vi "CRYCalc Arithmetic Unit&Ref.vi"(0 "A data for units":T1={"Name"="", "Curve"=[], "X data"=1, "Y data"=1, "Z data"=1, "X axis"=0, "Y axis"=1, "Z axis"=1, "X unit"="Hz", "Y unit"="", "Z unit"="deg.", "X dB ref"=1.0, "Y dB ref"=1.0, "Z dB ref"=1.0, "single val"=FALSE, "protected"=FALSE, "display X"=TRUE, "display Y"=TRUE, "display Z"=TRUE, "Test Info"="", "Step No."=0, "Plot Settings"={"Color"=0, "Interpolation"=0, "Point Style"=0, "Line Style"=0, "Point Color"=0, "Line Width"=0, "Bar Plot Style"=0, "Fill To"=0}, "AutoProtect"=FALSE} {"Z data" items=["dB", "Lin"]; "X data" items=["dB", "Lin"]; "Y data" items=["dB", "Lin"]; "Z dB ref" format="%.1f"; "Z axis" items=["Log", "Lin"]; "X dB ref" format="%.1f"; "X axis" items=["Log", "Lin"]; "Y axis" items=["Log", "Lin"]; "Y dB ref" format="%.1f"; "Curve"."z" format="%.2f"; "Curve"."y" format="%.2f"; "Curve"."x" format="%.2f"}, 5 "B data for units":T1={"Name"="", "Curve"=[], "X data"=1, "Y data"=1, "Z data"=1, "X axis"=0, "Y axis"=1, "Z axis"=1, "X unit"="Hz", "Y unit"="", "Z unit"="deg.", "X dB ref"=1.0, "Y dB ref"=1.0, "Z dB ref"=1.0, "single val"=FALSE, "protected"=FALSE, "display X"=TRUE, "display Y"=TRUE, "display Z"=TRUE, "Test Info"="", "Step No."=0, "Plot Settings"={"Color"=0, "Interpolation"=0, "Point Style"=0, "Line Style"=0, "Point Color"=0, "Line Width"=0, "Bar Plot Style"=0, "Fill To"=0}, "AutoProtect"=FALSE} {"Z data" items=["dB", "Lin"]; "X data" items=["dB", "Lin"]; "Y data" items=["dB", "Lin"]; "Z dB ref" format="%.1f"; "Z axis" items=["Log", "Lin"]; "X dB ref" format="%.1f"; "X axis" items=["Log", "Lin"]; "Y axis" items=["Log", "Lin"]; "Y dB ref" format="%.1f"; "Curve"."z" format="%.2f"; "Curve"."y" format="%.2f"; "Curve"."x" format="%.2f"}, 9 "operator":u16(ring) items=["+", "--", "x", "/"], 11 "Work in":u16(slide), 12 "Axis Mode":u16(slide)) -> (3 "Result X unit":string, 4 "Result Y unit":string, 6 "Result dB ref(A)":dbl=1.0 format="%.1f", 8 "Result Y data":u16, 10 "Single val out":bool, 14 "Result Z unit":string)   [LabVIEW 2013]
uses:
  Typedef Control/CRYData Cluster.ctl
  CRYPost Processing Global.vi
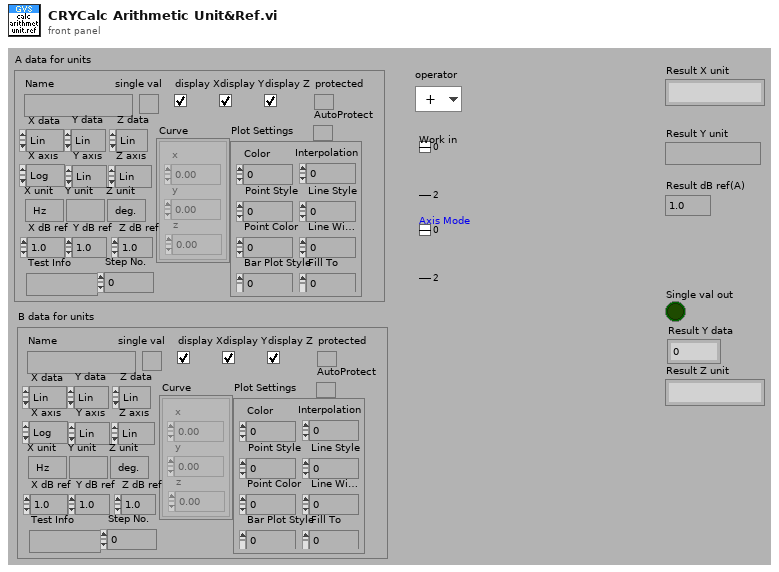
[diagram p1: front panel]
types:
  T1 = typedef "CRYData Cluster.ctl" = cluster{"Name":string, "Curve":cluster{"x":dbl, "y":dbl, "z":dbl}[], "X data":u16, "Y data":u16, "Z data":u16, "X axis":u16, "Y axis":u16, "Z axis":u16, "X unit":string, "Y unit":string, "Z unit":string, "X dB ref":dbl, "Y dB ref":dbl, "Z dB ref":dbl, "single val":bool, "protected":bool, "display X":bool, "display Y":bool, "display Z":bool, "Test Info":string, "Step No.":i32, "Plot Settings":cluster{"Color":u32, "Interpolation":u8, "Point Style":u8, "Line Style":u8, "Point Color":u32, "Line Width":u8, "Bar Plot Style":u8, "Fill To":i16}, "AutoProtect":bool}
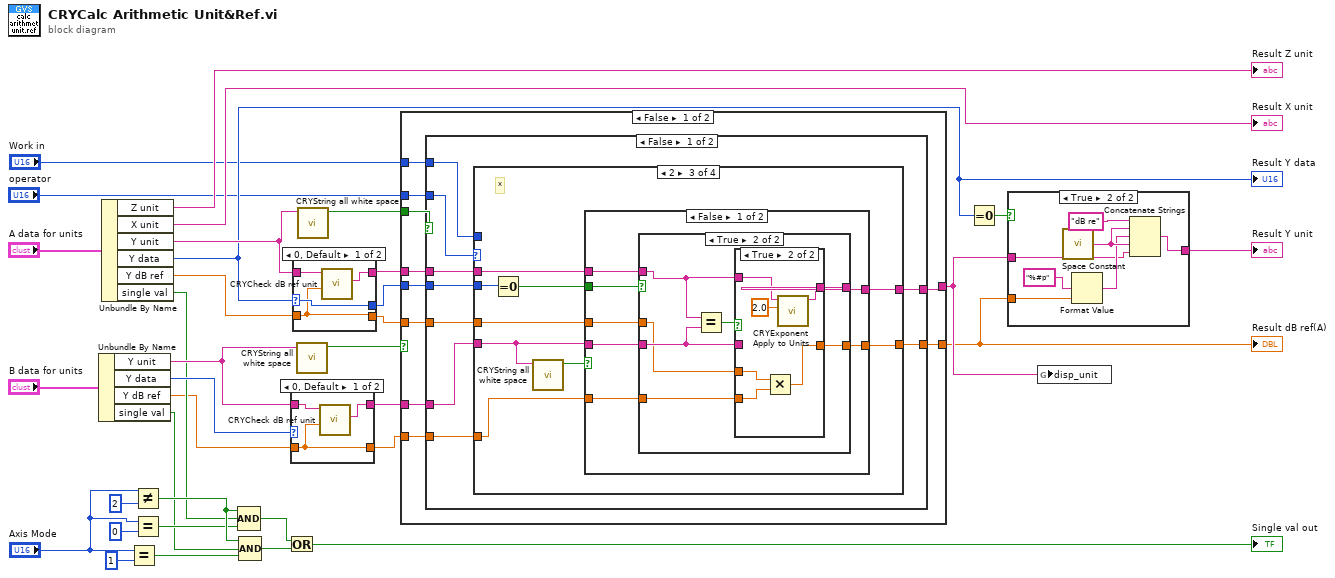
[diagram p0: block diagram]
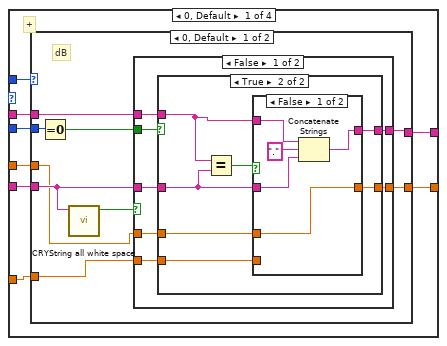
[diagram p2: hidden frame]
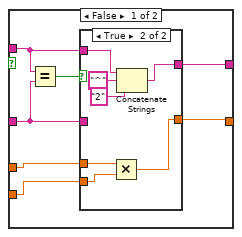
[diagram p3: hidden frame]
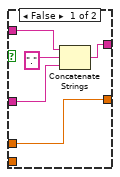
[diagram p4: hidden frame]
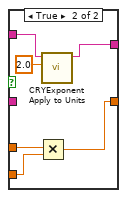
[diagram p5: hidden frame]
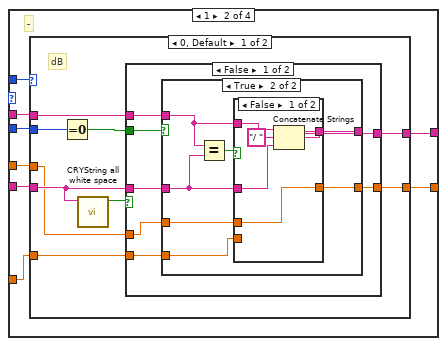
[diagram p8: hidden frame]
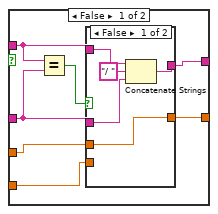
[diagram p9: hidden frame]
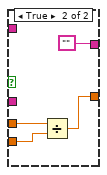
[diagram p10: hidden frame]
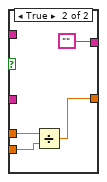
[diagram p11: hidden frame]
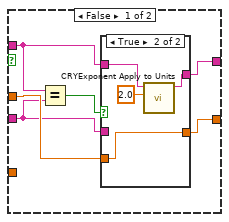
[diagram p14: hidden frame]
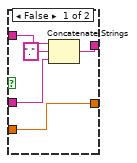
[diagram p15: hidden frame]
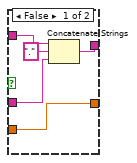
[diagram p16: hidden frame]
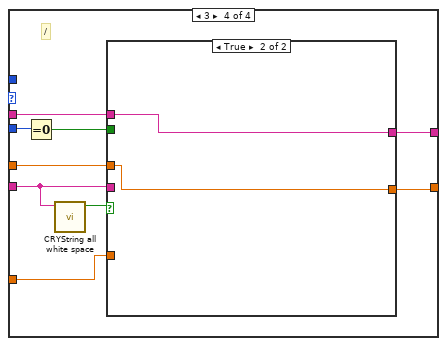
[diagram p18: hidden frame]
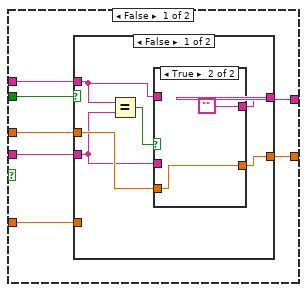
[diagram p19: hidden frame]
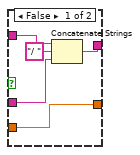
[diagram p20: hidden frame]
diagram:
  n1 = Unbundle By Name("B data for units") -> ("Y unit"=w35:string, "Y data"=w34:u16, "Y dB ref"=w17:dbl, "single val"=w21:bool)
  n2 = Unbundle By Name("A data for units") -> ("Z unit"=→"Result Z unit":string, "X unit"=→"Result X unit":string, "Y unit"=w14:string, "Y data"=w13:u16, "Y dB ref"=w12:dbl, "single val"=w22:bool)
  "Result Y data" <- w13
  n3 = Equal?(x="Axis Mode", y=u16 1) -> (x = y?=w28:bool)
  n4 = Not Equal?(x="Axis Mode", y=u16 2) -> (x != y?=w25:bool)
  n5 = Equal?(x="Axis Mode", y=u16 0) -> (x = y?=w23:bool)
  n6 = Compound Arithmetic op=AND(w25, w22, w23) -> (w26:bool)
  n7 = Compound Arithmetic op=AND(w25, w21, w28) -> (w27:bool)
  n8 = Or(x=w26, y=w27) -> (x .or. y?=→"Single val out":bool)
  n9 = case shown="0, Default" w34 {
    tunnel: w35 -> [w38 w40]
    tunnel: [w37 w40] -> w4
    tunnel: w17 -> [w36 w39]
    tunnel: [w36 w39] -> w1
    frame 0, Default {
      n10 = call "CRYCheck dB ref unit.vi"("dB ref in"=w36, "Unit in"=w38) -> ("Lin unit out"=w37:string)  [unwired: 9 out]
    }
    frame 1 {
    }
  }
  n11 = case shown="0, Default" w13 {
    selector: w13 -> [w42 w46]
    tunnel: w14 -> [w44 w47]
    tunnel: [w43 w47] -> w8
    tunnel: w12 -> [w41 w45]
    tunnel: [w42 w46] -> w7
    tunnel: [w41 w45] -> w6
    frame 0, Default {
      n12 = call "CRYCheck dB ref unit.vi"("dB ref in"=w41, "Unit in"=w44) -> ("Lin unit out"=w43:string)  [unwired: 9 out]
    }
    frame 1 {
    }
  }
  n13 = call "CRYString all white space.vi"("String"=w35) -> ("Nothing but white space?"=w5:bool)  [unwired: 10 in]
  n14 = call "CRYString all white space.vi"("String"=w14) -> ("Nothing but white space?"=w9:bool)  [unwired: 10 in]
  n15 = case shown="False" w5 {
    tunnel: [w57 w293] -> w3
    tunnel: w4 -> [w56 _]
    tunnel: w9 -> [w55 _]
    tunnel: w8 -> [w54 w293]
    tunnel: "Work in" -> [w53 _]
    tunnel: "operator" -> [w52 _]
    tunnel: w7 -> [w51 _]
    tunnel: w6 -> [w50 w292]
    tunnel: [w49 w292] -> w2
    tunnel: w1 -> [w48 _]
    frame False {
      n16 = case shown="False" w55 {
        tunnel: [w60 w291] -> w57
        tunnel: w56 -> [w63 w291]
        tunnel: w54 -> [w64 _]
        tunnel: w53 -> [w65 _]
        tunnel: w52 -> [w66 _]
        tunnel: w51 -> [w62 _]
        tunnel: w50 -> [w61 w290]
        tunnel: [w59 w290] -> w49
        tunnel: w48 -> [w58 _]
        frame False {
          n17 = case shown="2" w66 {
            tunnel: w65 -> [w74 w139 _ _]
            tunnel: w64 -> [w73 w138 w200 w251]
            tunnel: w63 -> [w72 w135 w196 w247]
            tunnel: w62 -> [w71 w137 w199 w250]
            tunnel: [w70 w134 w198 w249] -> w60
            tunnel: w61 -> [w69 w136 w194 w245]
            tunnel: [w68 w133 w192 w243] -> w59
            tunnel: w58 -> [w67 w132 w193 w244]
            frame 0, Default {
              # "+"
              n18 = case shown="0, Default" w74 {
                tunnel: w73 -> [w82 w131]
                tunnel: w72 -> [w79 _]
                tunnel: w71 -> [w83 _]
                tunnel: [w81 w131] -> w70
                tunnel: w69 -> [w76 w130]
                tunnel: [w75 w130] -> w68
                tunnel: w67 -> [w77 _]
                frame 0, Default {
                  # "dB"
                  n19 = Equal To 0?(x=w83) -> (x = 0?=w80:bool)
                  n20 = call "CRYString all white space.vi"("String"=w79) -> ("Nothing but white space?"=w78:bool)  [unwired: 10 in]
                  n21 = case shown="False" w78 {
                    tunnel: w82 -> [w90 w129]
                    tunnel: [w89 w129] -> w81
                    tunnel: w80 -> [w88 _]
                    tunnel: w79 -> [w87 _]
                    tunnel: w77 -> [w86 _]
                    tunnel: w76 -> [w85 w128]
                    tunnel: [w84 w128] -> w75
                    frame False {
                      n22 = case shown="True" w88 {
                        tunnel: w90 -> [w96 w113]
                        tunnel: w87 -> [w94 w114]
                        tunnel: [w95 w115] -> w89
                        tunnel: w86 -> [w92 w111]
                        tunnel: w85 -> [w93 w112]
                        tunnel: [w91 w110] -> w84
                        frame False {
                          n23 = Equal?(x=w96, y=w94) -> (x = y?=w97:bool)
                          n24 = case shown="True" w97 {
                            tunnel: w96 -> [w102 w109]
                            tunnel: [w99 w106] -> w95
                            tunnel: w94 -> [w100 _]
                            tunnel: w93 -> [w98 w105]
                            tunnel: w92 -> [_ w104]
                            tunnel: [w98 w103] -> w91
                            frame False {
                              n25 = Concatenate Strings(w102, "." ("string"), w100) -> (w99:string)
                            }
                            frame True {
                              n26 = Multiply(x=w105, y=w104) -> (x*y=w103:dbl)
                              n27 = Concatenate Strings(w109, "^" ("string"), "2" ("string")) -> (w106:string)
                            }
                          }
                        }
                        frame True {
                          n28 = Equal?(x=w113, y=w114) -> (x = y?=w116:bool)
                          n29 = case shown="False" w116 {
                            tunnel: w113 -> [w119 w126]
                            tunnel: [w118 w125] -> w115
                            tunnel: w114 -> [w120 _]
                            tunnel: w112 -> [w117 w124]
                            tunnel: w111 -> [_ w123]
                            tunnel: [w117 w122] -> w110
                            frame False {
                              n30 = Concatenate Strings(w119, "." ("string"), w120) -> (w118:string)
                            }
                            frame True {
                              n31 = Multiply(x=w124, y=w123) -> (x*y=w122:dbl)
                              n32 = call "CRYExponent Apply to Units.vi"("Exponent to apply"=2.0, "Unit in"=w126) -> ("Unit out"=w125:string)  [unwired: 9 out]
                            }
                          }
                        }
                      }
                    }
                    frame True {
                    }
                  }
                }
                frame 1, 2 {
                }
              }
            }
            frame 1 {
              # "-"
              n33 = case shown="0, Default" w139 {
                tunnel: w138 -> [w147 w191]
                tunnel: w135 -> [w144 _]
                tunnel: w137 -> [w148 _]
                tunnel: [w146 w191] -> w134
                tunnel: w136 -> [w142 w190]
                tunnel: [w140 w190] -> w133
                tunnel: w132 -> [w141 _]
                frame 0, Default {
                  # "dB"
                  n34 = Equal To 0?(x=w148) -> (x = 0?=w145:bool)
                  n35 = call "CRYString all white space.vi"("String"=w144) -> ("Nothing but white space?"=w143:bool)  [unwired: 10 in]
                  n36 = case shown="False" w143 {
                    tunnel: w147 -> [w155 w189]
                    tunnel: [w154 w189] -> w146
                    tunnel: w145 -> [w153 _]
                    tunnel: w144 -> [w152 _]
                    tunnel: w142 -> [w151 w188]
                    tunnel: w141 -> [w150 _]
                    tunnel: [w149 w188] -> w140
                    frame False {
                      n37 = case shown="True" w153 {
                        tunnel: w155 -> [w161 w175]
                        tunnel: w152 -> [w160 w176]
                        tunnel: [w159 w177] -> w154
                        tunnel: w151 -> [w158 w174]
                        tunnel: w150 -> [w157 w173]
                        tunnel: [w156 w172] -> w149
                        frame False {
                          n38 = Equal?(x=w161, y=w160) -> (x = y?=w162:bool)
                          n39 = case shown="False" w162 {
                            tunnel: w161 -> [w166 _]
                            tunnel: [w167 ""] -> w159
                            tunnel: w160 -> [w164 _]
                            tunnel: w158 -> [w163 w170]
                            tunnel: w157 -> [_ w169]
                            tunnel: [w163 w168] -> w156
                            frame False {
                              n40 = Concatenate Strings(w166, "/ " ("string"), w164) -> (w167:string)
                            }
                            frame True {
                              n41 = Divide(x=w170, y=w169) -> (x/y=w168:dbl)
                            }
                          }
                        }
                        frame True {
                          n42 = Equal?(x=w175, y=w176) -> (x = y?=w178:bool)
                          n43 = case shown="False" w178 {
                            tunnel: w175 -> [w182 _]
                            tunnel: [w183 ""] -> w177
                            tunnel: w176 -> [w180 _]
                            tunnel: w174 -> [w179 w186]
                            tunnel: w173 -> [_ w185]
                            tunnel: [w179 w184] -> w172
                            frame False {
                              n44 = Concatenate Strings(w182, "/ " ("string"), w180) -> (w183:string)
                            }
                            frame True {
                              n45 = Divide(x=w186, y=w185) -> (x/y=w184:dbl)
                            }
                          }
                        }
                      }
                    }
                    frame True {
                    }
                  }
                }
                frame 1, 2 {
                }
              }
            }
            frame 2 {
              # "*"
              n46 = Equal To 0?(x=w199) -> (x = 0?=w197:bool)
              n47 = call "CRYString all white space.vi"("String"=w196) -> ("Nothing but white space?"=w195:bool)  [unwired: 10 in]
              n48 = case shown="False" w195 {
                tunnel: w200 -> [w207 w242]
                tunnel: [w206 w242] -> w198
                tunnel: w197 -> [w205 _]
                tunnel: w196 -> [w204 _]
                tunnel: w194 -> [w203 w241]
                tunnel: w193 -> [w202 _]
                tunnel: [w201 w241] -> w192
                frame False {
                  n49 = case shown="True" w205 {
                    tunnel: w207 -> [w212 w226]
                    tunnel: w204 -> [w208 w227]
                    tunnel: [w211 w228] -> w206
                    tunnel: w203 -> [w210 w225]
                    tunnel: w202 -> [_ w224]
                    tunnel: [w209 w223] -> w201
                    frame False {
                      n50 = Equal?(x=w212, y=w208) -> (x = y?=w213:bool)
                      n51 = case shown="True" w213 {
                        tunnel: w212 -> [w217 w221]
                        tunnel: [w218 w220] -> w211
                        tunnel: w208 -> [w214 _]
                        tunnel: w210 -> [w215 w219]
                        tunnel: [w215 w219] -> w209
                        frame False {
                          n52 = Concatenate Strings(w217, "." ("string"), w214) -> (w218:string)
                        }
                        frame True {
                          n53 = call "CRYExponent Apply to Units.vi"("Exponent to apply"=2.0, "Unit in"=w221) -> ("Unit out"=w220:string)  [unwired: 9 out]
                        }
                      }
                    }
                    frame True {
                      n54 = Equal?(x=w226, y=w227) -> (x = y?=w229:bool)
                      n55 = case shown="True" w229 {
                        tunnel: w226 -> [w233 w239]
                        tunnel: [w234 w238] -> w228
                        tunnel: w227 -> [w231 _]
                        tunnel: w225 -> [w230 w237]
                        tunnel: w224 -> [_ w236]
                        tunnel: [w230 w235] -> w223
                        frame False {
                          n56 = Concatenate Strings(w233, "." ("string"), w231) -> (w234:string)
                        }
                        frame True {
                          n57 = Multiply(x=w237, y=w236) -> (x*y=w235:dbl)
                          n58 = call "CRYExponent Apply to Units.vi"("Exponent to apply"=2.0, "Unit in"=w239) -> ("Unit out"=w238:string)  [unwired: 9 out]
                        }
                      }
                    }
                  }
                }
                frame True {
                }
              }
            }
            frame 3 {
              # "/"
              n59 = Equal To 0?(x=w250) -> (x = 0?=w248:bool)
              n60 = call "CRYString all white space.vi"("String"=w247) -> ("Nothing but white space?"=w246:bool)  [unwired: 10 in]
              n61 = case shown="True" w246 {
                tunnel: w251 -> [w258 w289]
                tunnel: [w257 w289] -> w249
                tunnel: w248 -> [w256 _]
                tunnel: w247 -> [w255 _]
                tunnel: w245 -> [w254 w288]
                tunnel: w244 -> [w253 _]
                tunnel: [w252 w288] -> w243
                frame False {
                  n62 = case shown="False" w256 {
                    tunnel: w258 -> [w260 w275]
                    tunnel: w255 -> [w259 w276]
                    tunnel: [w261 w277] -> w257
                    tunnel: w254 -> [w263 w273]
                    tunnel: w253 -> [_ w274]
                    tunnel: [w262 w272] -> w252
                    frame False {
                      n63 = Equal?(x=w260, y=w259) -> (x = y?=w264:bool)
                      n64 = case shown="True" w264 {
                        tunnel: w260 -> [w268 _]
                        tunnel: [w269 ""] -> w261
                        tunnel: w259 -> [w266 _]
                        tunnel: w263 -> [w265 w270]
                        tunnel: [w265 w270] -> w262
                        frame False {
                          n65 = Concatenate Strings(w268, "/ " ("string"), w266) -> (w269:string)
                        }
                        frame True {
                        }
                      }
                    }
                    frame True {
                      n66 = Equal?(x=w275, y=w276) -> (x = y?=w278:bool)
                      n67 = case shown="False" w278 {
                        tunnel: w275 -> [w282 _]
                        tunnel: [w283 ""] -> w277
                        tunnel: w276 -> [w280 _]
                        tunnel: w274 -> [_ w285]
                        tunnel: w273 -> [w279 w286]
                        tunnel: [w279 w284] -> w272
                        frame False {
                          n68 = Concatenate Strings(w282, "/ " ("string"), w280) -> (w283:string)
                        }
                        frame True {
                          n69 = Divide(x=w286, y=w285) -> (x/y=w284:dbl)
                        }
                      }
                    }
                  }
                }
                frame True {
                }
              }
            }
          }
        }
        frame True {
        }
      }
    }
    frame True {
    }
  }
  "Result dB ref(A)" <- w2
  n70 = Equal To 0?(x=w13) -> (x = 0?=w16:bool)
  n71 = case shown="True" w16 {
    tunnel: w3 -> [w294 w296]
    tunnel: [w294 w295] -> w15
    tunnel: w2 -> [_ w300]
    frame False {
    }
    frame True {
      n72 = call <vilib>:"Space Constant.vi"() -> ("String"=w299:string)
      n73 = Format Value(format string="%#p", value (0)=w300) -> (output string=w297:string)  [unwired: 1 out]
      n74 = Concatenate Strings("dB re" ("string"), w299, w297, w299, w296) -> (w295:string)
    }
  }
  "Result Y unit" <- w15
  n75 = global write "CRYPost Processing Global.vi" "disp_unit"(w3) -> ()
